vi "OpenSwerveDrive.vi"(6 "error in":errorcluster, 7 "Ramp Rate":dbl, 8 "Speed PID":cluster{"P":dbl, "I":dbl, "D":dbl}, 9 "Steering PID":cluster{"P":dbl, "I":dbl, "D":dbl}) -> (0 "error out":errorcluster)   [LabVIEW 2014]
uses:
  <vilib>/Rock Robotics/WPI/CAN/TalonSRX/WPI_CANTalonSRX_APIControlMode.ctl
  <vilib>/Rock Robotics/WPI/CAN/TalonSRX/WPI_CANTalonSRX_APIFeedbackSelect.ctl
  <vilib>/Rock Robotics/WPI/MotorControl/WPI_MotorControlOpenCANTalonSRX.vi
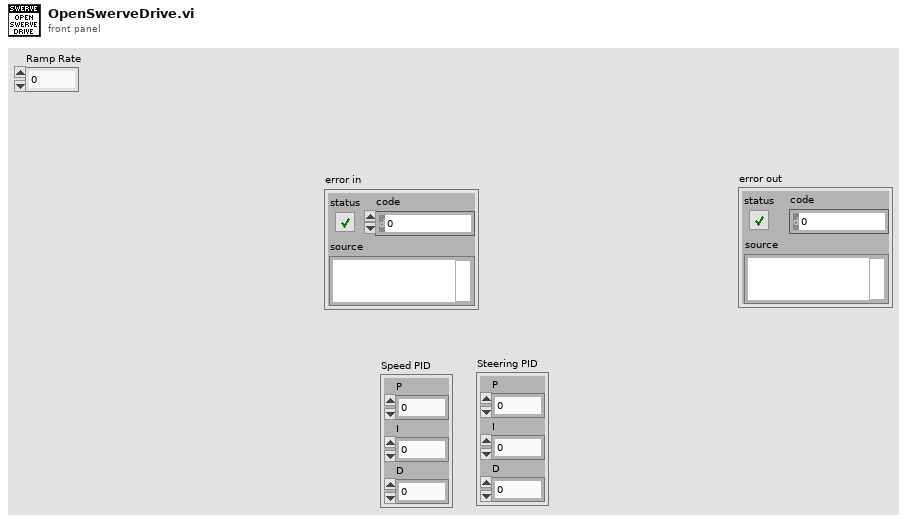
[diagram p1: front panel]
types:
  T1 = typedef "WPI_CANTalonSRX_APIControlMode.ctl" = enum8{"Percent VBus", "Speed", "Position", "Slave", "Unchanged / Invalid"}
  T2 = typedef "WPI_CANTalonSRX_APIFeedbackSelect.ctl" = enum16{"Digital Quadrature Encoder", "Analog Potentiometer", "Analog Encoder"}
  T3 = typedef "WPI_MotorControlDeviceRef.ctl" = cluster{"DeviceStatus":errorcluster, "Type":T4, "PWM":cluster{"Controller":T5, "PWM Channel":T6, "DeadBand":T7}, "CAN":cluster{"Device Number":u8, "Control Mode":T8, "Semaphore":T9, "Max Vout":dbl, "TalonSRX Control Mode":T1}, "Invert":bool, "TransformRef":T10, "InvTransformRef":T10}
  T4 = typedef "WPI_MotorControlType.ctl" = enum16{"PWM", "CAN", "CANTalonSRX"}
  T5 = typedef "FPGA_TypedefDigitalModule.ctl" = enum16{"Controller 1"}
  T6 = typedef "FPGA_DIOPWMChannel.ctl" = enum8{"PWM 0", "PWM 1", "PWM 2", "PWM 3", "PWM 4", "PWM 5", "PWM 6", "PWM 7", "PWM 8", "PWM 9", "PWM MXP 0", "PWM MXP 1", "PWM MXP 2", "PWM MXP 3", "PWM MXP 4", "PWM MXP 5", "PWM MXP 6", "PWM MXP 7", "PWM MXP 8", "PWM MXP 9", "Invalid"}
  T7 = typedef "WPI_PWMDeadband.ctl" = cluster{"Name":string, "maxPositivePwm":i32, "minPositivePwm":i32, "centerPwm":i32, "maxNegativePwm":i32, "minNegativePwm":i32, "angularRange":u16}
  T8 = typedef "WPI_CANJaguar_ControlMode.ctl" = enum8{"Percent VBus", "Current", "Speed", "Position", "Voltage"}
  T9 = typedef "Semaphore RefNum" = refnum<k1>
  T10 = typedef "WPI_PWMTransform_ConPane.ctl" = refnum<vi>
  T11 = typedef "WPI_CANTalonSRX_GlobalStatus.ctl" = cluster{"Applied Throttle":dbl, "Module Enabled":bool, "CAN Error":errorcluster, "Closed Loop Error":dbl, "Forward Limit Switch Closed":bool, "Reverse Limit Switch Closed":bool, "Sensor Position":dbl, "Sensor Velocity":dbl, "Current":dbl, "Sticky Fault - Over Temp":bool, "Sticky Fault - Under Voltage":bool, "Sticky Fault - Forward Limit":bool, "Sticky Fault - Reverse Limit":bool, "Sticky Fault - Forward Soft Limit":bool, "Sticky Fault - Reverse Soft Limit":bool, "Brake is Enabled":bool, "Encoder Position":dbl, "Encoder Velocity":dbl, "Encoder Index Count":dbl, "Encoder A Pin State":bool, "Encoder B Pin State":bool, "Encoder Index Pin State":bool, "Analog In":dbl, "Analog In Velocity":dbl, "Temperature (C)":dbl, "Battery Voltage":dbl}
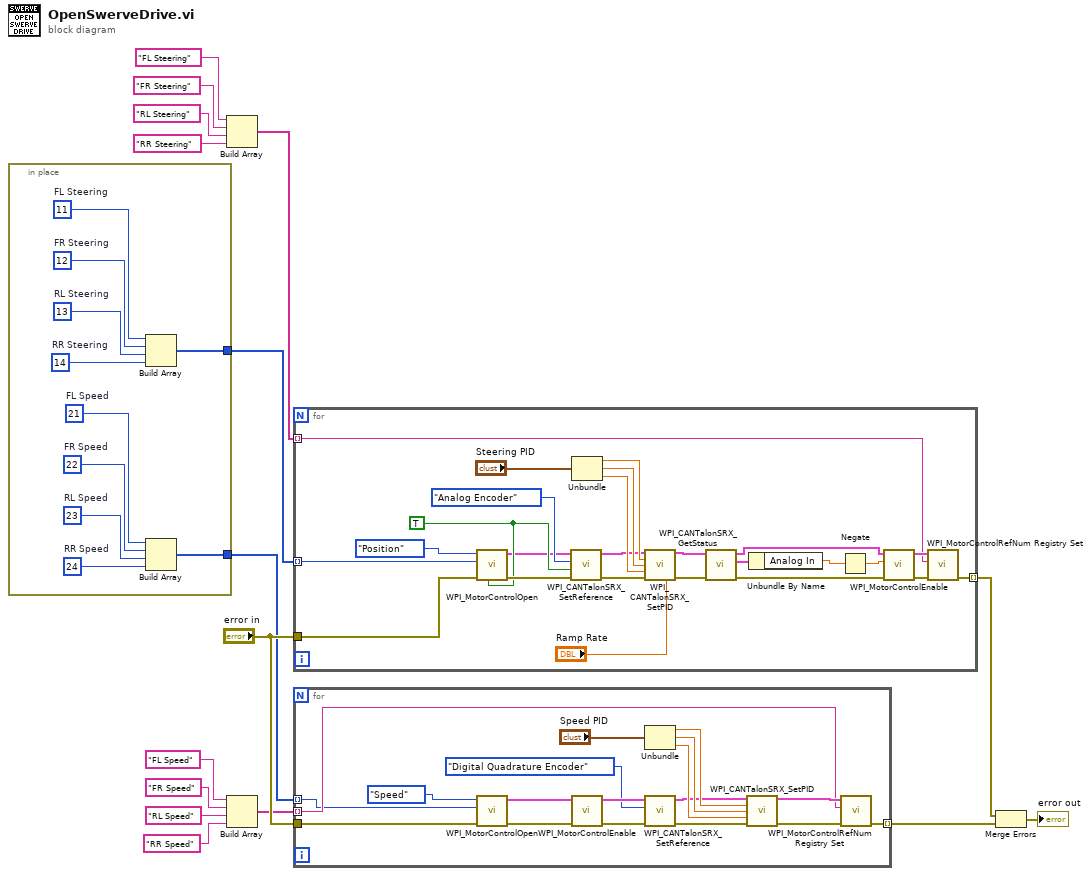
[diagram p0: block diagram]
diagram:
  n1 = in-place {
    in-place-border: [w22] -> w13
    in-place-border: [w17] -> w1
    w26 = u8 11  # FL Steering
    w18 = u8 24  # RR Speed
    w19 = u8 23  # RL Speed
    w20 = u8 22  # FR Speed
    w21 = u8 21  # FL Speed
    w23 = u8 14  # RR Steering
    w24 = u8 13  # RL Steering
    w25 = u8 12  # FR Steering
    n2 = Build Array(w26, w25, w24, w23) -> (w22:u8[])
    n3 = Build Array(w21, w20, w19, w18) -> (w17:u8[])
  }
  n4 = Build Array("FL Steering" ("refnum name"), "FR Steering" ("refnum name"), "RL Steering" ("refnum name"), "RR Steering" ("refnum name")) -> (w8:string[])
  n5 = Build Array("FL Speed" ("refnum name"), "FR Speed" ("refnum name"), "RL Speed" ("refnum name"), "RR Speed" ("refnum name")) -> (w2:string[])
  n6 = for {
    tunnel: "error in" -> [w48]
    tunnel: [w43] -> w7 mode=indexing
    tunnel: w13 -> [w38] mode=indexing
    tunnel: w8 -> [w37] mode=indexing
    w34 = TRUE ("Invert")
    n7 = call-poly <vilib>:"WPI_MotorControlOpen.vi"("Invert"=w34, "error in (no error)"=w48, "Device Number"=w38, "Control Mode"=WPI_CANTalonSRX_APIControlMode."Position") -> ("error out"=w44:errorcluster, "MotorControlDeviceRef"=w28:T3)  [unwired: 6 in]
    n8 = call <vilib>:"WPI_CANTalonSRX_SetReference.vi"("error in (no error)"=w44, "Reverse Feedback Sensor"=w34, "Feedback Reference"=WPI_CANTalonSRX_APIFeedbackSelect."Analog Encoder", "CAN Talon SRX Ref"=w28) -> ("error out"=w47:errorcluster, "CAN Talon SRX Ref Out"=w46:T3)  [unwired: 6 in]
    n9 = Unbundle("Steering PID") -> ("P"=w51:dbl, "I"=w50:dbl, "D"=w49:dbl)
    n10 = call <vilib>:"WPI_CANTalonSRX_SetPID.vi"("CAN Talon SRX Ref"=w46, "P"=w51, "I"=w50, "D"=w49, "error in (no error)"=w47, "Ramp Rate"="Ramp Rate") -> ("CAN Talon SRX Ref Out"=w42:T3, "error out"=w39:errorcluster)  [unwired: 8 in]
    n11 = call <vilib>:"WPI_CANTalonSRX_GetStatus.vi"("error in (no error)"=w39, "CAN Talon SRX Ref"=w42) -> ("error out"=w29:errorcluster, "Talon SRX Status"=w32:T11, "CAN Talon SRX Ref Out"=w33:T3)  [unwired: 7 in]
    n12 = Unbundle By Name(w32) -> ("Analog In"=w31:dbl)
    n13 = Negate(x=w31) -> (-x=w30:dbl)
    n14 = call <vilib>:"WPI_MotorControlEnable.vi"("error in (no error)"=w29, "Encoder Initial Position"=w30, "CAN Jaguar Ref"=w33) -> ("error out"=w40:errorcluster, "CAN Jaguar Ref Out"=w41:T3)  [unwired: 7 in]
    n15 = call <vilib>:"WPI_MotorControlRefNum Registry Set.vi"("error in (no error)"=w40, "refnum name"=w37, "MotorControlDevRef"=w41) -> ("error out"=w43:errorcluster)  [unwired: 7 in, 1 out]
  }
  n16 = for {
    tunnel: "error in" -> [w65]
    tunnel: [w62] -> w15 mode=indexing
    tunnel: w2 -> [w53] mode=indexing
    tunnel: w1 -> [w52] mode=indexing
    n17 = call-poly <vilib>:"WPI_MotorControlOpen.vi"("error in (no error)"=w65, "Device Number"=w52, "Control Mode"=WPI_CANTalonSRX_APIControlMode."Speed") -> ("error out"=w56:errorcluster, "MotorControlDeviceRef"=w55:T3)  [unwired: 7 in]
    n18 = call <vilib>:"WPI_MotorControlEnable.vi"("error in (no error)"=w56, "CAN Jaguar Ref"=w55) -> ("error out"=w59:errorcluster, "CAN Jaguar Ref Out"=w58:T3)  [unwired: 8 in]
    n19 = Unbundle("Speed PID") -> ("P"=w68:dbl, "I"=w67:dbl, "D"=w66:dbl)
    n20 = call <vilib>:"WPI_CANTalonSRX_SetReference.vi"("error in (no error)"=w59, "Feedback Reference"=WPI_CANTalonSRX_APIFeedbackSelect."Digital Quadrature Encoder", "CAN Talon SRX Ref"=w58) -> ("error out"=w60:errorcluster, "CAN Talon SRX Ref Out"=w61:T3)  [unwired: 7 in]
    n21 = call <vilib>:"WPI_CANTalonSRX_SetPID.vi"("CAN Talon SRX Ref"=w61, "P"=w68, "I"=w67, "D"=w66, "error in (no error)"=w60) -> ("CAN Talon SRX Ref Out"=w63:T3, "error out"=w64:errorcluster)  [unwired: 9 in]
    n22 = call <vilib>:"WPI_MotorControlRefNum Registry Set.vi"("error in (no error)"=w64, "refnum name"=w53, "MotorControlDevRef"=w63) -> ("error out"=w62:errorcluster)  [unwired: 7 in, 1 out]
  }
  n23 = Merge Errors(w7, w15) -> (→"error out":errorcluster)
